vi "Initialize.vi"(8 "error in (no error)":errorcluster, 11 "Relay-Box in":refnum<class "Relay-Box.lvclass">) -> (0 "error out":errorcluster, 3 "Relay-Box out":refnum<class "Relay-Box.lvclass">)   [LabVIEW 2019, in "Relay-Box.lvclass"]
uses:
  <userlib>/LevyLab/Relay Box/Relay-Box.lvclass
  <userlib>/LevyLab/Relay Box/Relay-Box.lvclass/Relay-Box.ctl
  <userlib>/LevyLab/Relay Box/D2XX_Functions/D2XX_Functions.lvlib
panel:
  out "FT_Status":u32(ring) items=["FT_OK", "FT_INVALID_HANDLE", "FT_DEVICE_NOT_FOUND", "FT_DEVICE_NOT_OPENED", "FT_IO_ERROR", "FT_INSUFFICIENT_RESOURCES", "FT_INVALID_PARAMETER", "FT_INVALID_BAUD_RATE", "FT_DEVICE_NOT_OPENED_FOR_ERASE", "FT_DEVICE_NOT_OPENED_FOR_WRITE", "FT_FAILED_TO_WRITE_DEVICE", "FT_EEPROM_READ_FAILED", "FT_EEPROM_WRITE_FAILED", "FT_EEPROM_ERASE_FAILED", "FT_EEPROM_NOT_PRESENT", "FT_EEPROM_NOT_PROGRAMMED", "FT_INVALID_ARGS", "FT_NOT_SUPPORTED", "FT_OTHER_ERROR"]
  out "Port Index":string
  out "Device Description":string
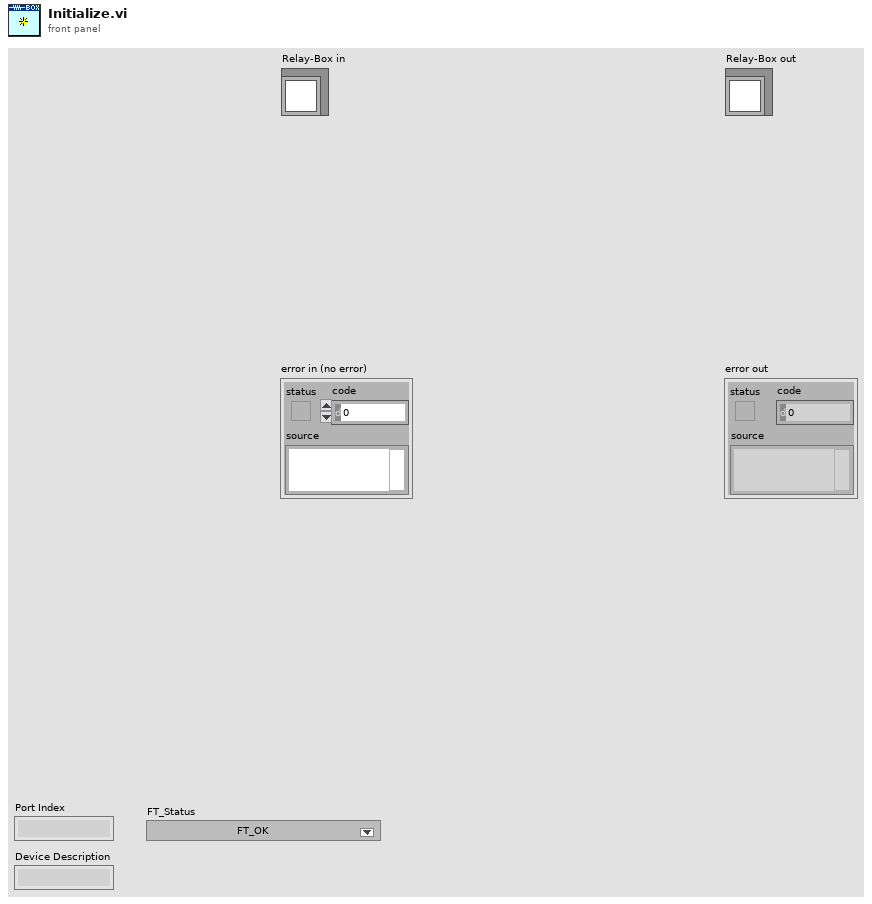
[diagram p1: front panel]
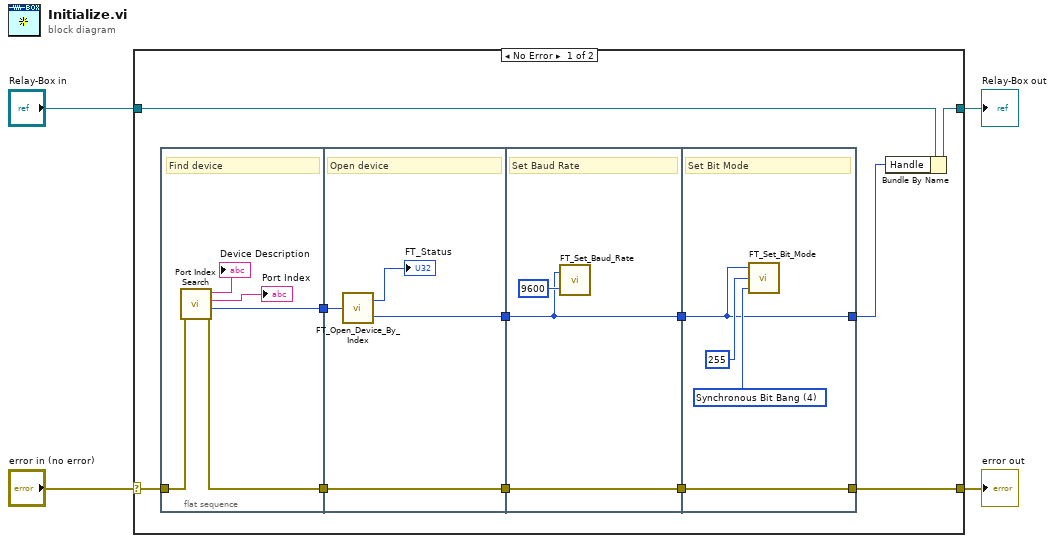
[diagram p0: block diagram]
diagram:
  n1 = case shown="No Error" "error in (no error)" {
    selector: "error in (no error)" -> [w7 w33]
    tunnel: [w6 w33] -> w3
    tunnel: [w15 w32] -> w1
    tunnel: "Relay-Box in" -> [w14 w32]
    frame No Error {
      n2 = flat-sequence {
        tunnel: [w19] -> w13
        tunnel: w7 -> [w17]
        tunnel: [w18] -> w12
        tunnel: w13 -> [w23]
        tunnel: [w21] -> w11
        tunnel: [w22] -> w10
        tunnel: w12 -> [w22]
        tunnel: [w25] -> w9
        tunnel: w11 -> [w25]
        tunnel: [w26] -> w8
        tunnel: w10 -> [w26]
        tunnel: w9 -> [w28]
        tunnel: w8 -> [w29]
        tunnel: [w29] -> w6
        tunnel: [w28] -> w5
        frame #0 {
          # "Find device"
          n3 = call <userlib>:"Port Index Search.vi"("error in"=w17) -> ("error out"=w18:errorcluster, "Decimal Port Index"=w19:i32, "Port Index"=→"Port Index":string, "Device Description"=→"Device Description":string)  [unwired: 7 in]
        }
        frame #1 {
          # "Open device"
          n4 = call <userlib>:"FT_Open_Device_By_Index.vi"("Device Index"=w23) -> ("FT_Status"=→"FT_Status":u32, "Handle"=w21:u32)
        }
        frame #2 {
          # "Set Baud Rate"
          n5 = call <userlib>:"FT_Set_Baud_Rate.vi"("Baud Rate"=u32 9600, "Handle"=w25) -> ()  [unwired: 1 out]
        }
        frame #3 {
          w30 = u8 4 items=["Reset Bit Mode"=0, "Asynchronous Bit Bang"=1, "MPSSE"=2, "Synchronous Bit Bang"=4, "MCU Host Bus Emulation"=8, "Fast Opto-Isolated Serial"=16, "CBUS Bit Bang"=32, "Single Channel 245 Synchronous FIFO"=64] ("Bit Mode")
          # "Set Bit Mode"
          n6 = call <userlib>:"FT_Set_Bit_Mode.vi"("Bit Mode"=w30, "Bit Mode Mask"=u8 255, "Handle"=w28) -> ()  [unwired: 1 out]
        }
      }
      n7 = Bundle By Name(cluster=w14, "Handle"=w5) -> (w15:refnum<class "Relay-Box.lvclass">)
    }
    frame Error {
    }
  }
  "error out" <- w3
  "Relay-Box out" <- w1
